vi "Read CallerParameter.vi"(8 "error in (no error)":errorcluster, 11 "AsynchReturnMsg in":refnum<class "CS++AsynchReturnMsg.lvclass">) -> (0 "error out":errorcluster, 2 "CallerParameter":variant, 3 "AsynchReturnMsg out":refnum<class "CS++AsynchReturnMsg.lvclass">)   [LabVIEW 2015, in "CS++AsynchReturnMsg.lvlib" / "CS++AsynchReturnMsg.lvclass"]
uses:
  CS++AsynchReturnMsg.lvclass
  CS++AsynchReturnMsg.lvclass/CS++AsynchReturnMsg.ctl
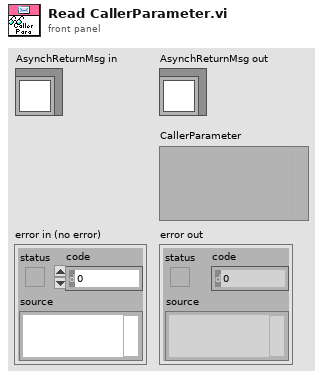
[diagram p1: front panel]
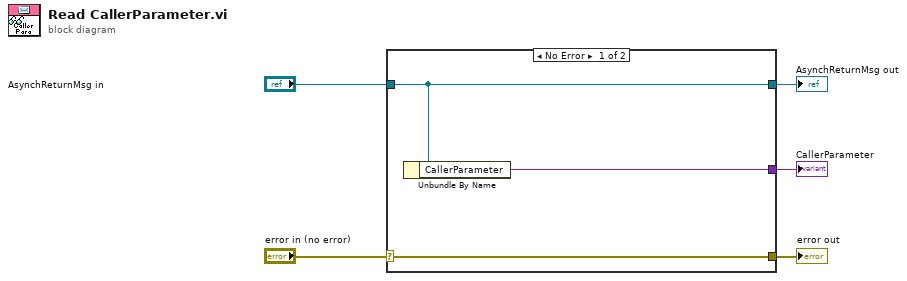
[diagram p0: block diagram]
diagram:
  n1 = case shown="No Error" "error in (no error)" {
    selector: "error in (no error)" -> [w8 w9]
    tunnel: [w8 w9] -> w4
    tunnel: [w7 w10] -> w2
    tunnel: "AsynchReturnMsg in" -> [w7 w10]
    tunnel: [w6 _] -> w1
    frame No Error {
      n2 = Unbundle By Name(w7) -> ("CallerParameter"=w6:variant)
    }
    frame Error {
    }
  }
  "error out" <- w4
  "AsynchReturnMsg out" <- w2
  "CallerParameter" <- w1
